vi "Run.vi"   [LabVIEW 2010, in "BehaviorClassification.lvclass"]
uses:
  BehaviorClassification.lvclass
  TrialBasedExperimentObject/TrialBasedExperiment.lvclass
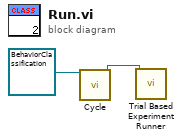
[diagram p0: block diagram]
diagram:
  n1 = call-dynamic "Cycle.vi"("BehaviorClassification In"=refnum<class "BehaviorClassification.lvclass"> refnum ("BehaviorClassification.lvclass")) -> ("BehaviorClassification Out"=w1:refnum<class "BehaviorClassification.lvclass">)  [unwired: 9 in, 1 out]
  n2 = call "Trial Based Experiment Runner.vi"(11:w1) -> ()  [unwired: 11 in]
